vi "Add Channel Properties To String Array.vi"(8 "error in":errorcluster, 10 "Properties List In":string[][](array[string]), 11 "Channel Ref in":T1 format="%.0x") -> (0 "error out":errorcluster, 2 "Properties List Out":string[][](array[string]), 3 "Channel Ref out":T1 format="%.0x")   [LabVIEW 2026, in "SEECD System Explorer.lvlib"]
uses:
  SEECD System Explorer.lvlib
  <vilib>/NI VeriStand/Custom Device API/Custom Device Item Ref.ctl
  Shared/Type Defs/ECAT Channel Data Type.ctl
  <vilib>/Utility/error.llb/Trim Whitespace One-Sided.vi
  C:/Users/Administrator/Desktop/Jatin/All DNC DLLs/NationalInstruments.VeriStand.SystemDefinitionAPI.dll
  Jatin/All DNC DLLs/NationalInstruments.VeriStand.SystemDefinitionAPI.dll
  Shared/Globals/Property Strings.vi
  C:/Users/Administrator/Desktop/Jatin/All DNC DLLs/NationalInstruments.VeriStand.SystemStorage.dll
  Jatin/All DNC DLLs/NationalInstruments.VeriStand.SystemStorage.dll
  Shared/SEECD Shared.lvlib
  <vilib>/NI VeriStand/Custom Device API/Custom Device API.lvlib
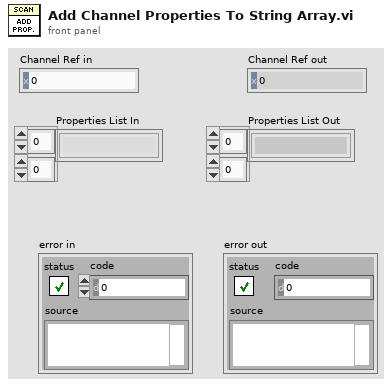
[diagram p1: front panel]
types:
  T1 = typedef "Custom Device API.lvlib/Custom Device Item Ref.ctl" = u64
  T2 = typedef "SEECD Shared.lvlib/ECAT Channel Data Type.ctl" = enum16{"Boolean", "Fixed Point", "Int8", "Int16", "Int32", "Int64", "U32 Bit Field", "UInt8", "UInt16", "UInt32", "UInt64", "Other", "DBL", "SGL"}
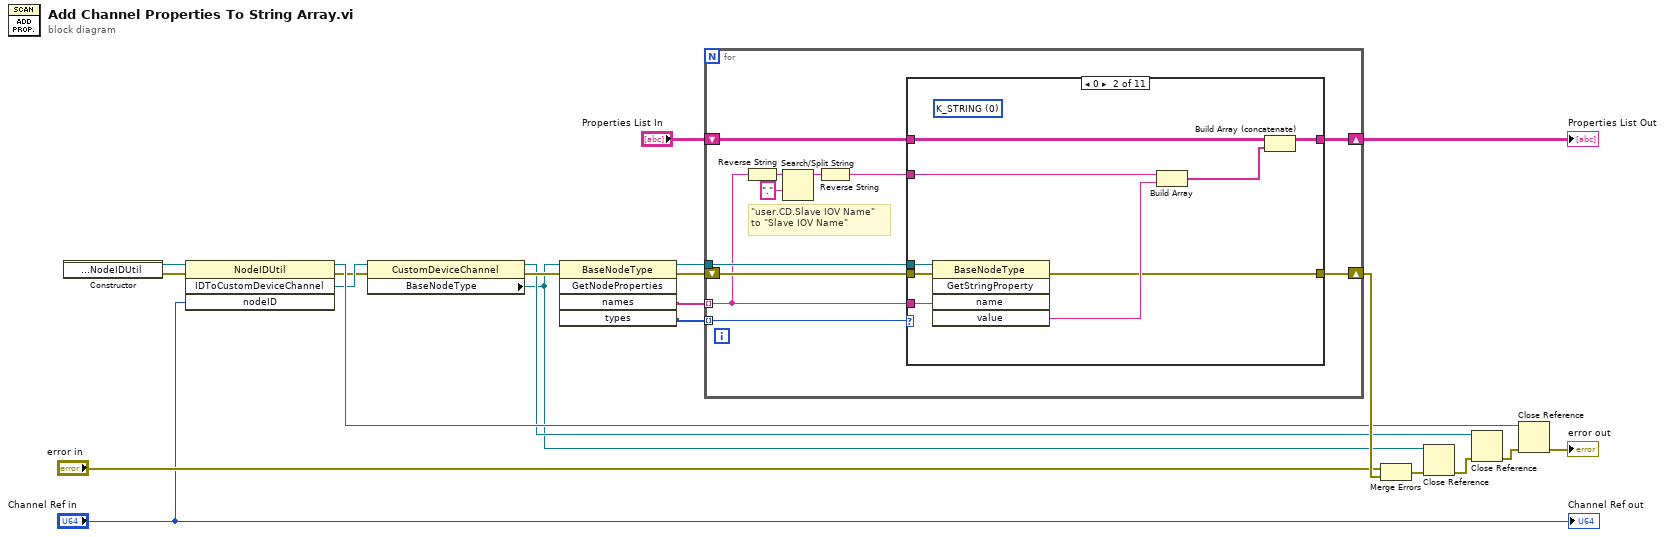
[diagram p0: block diagram]
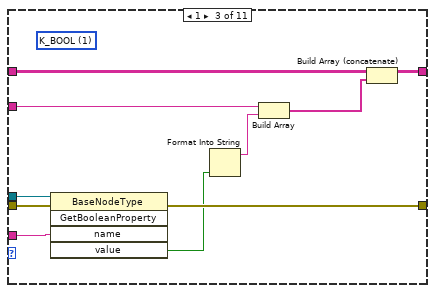
[diagram p3: hidden frame]
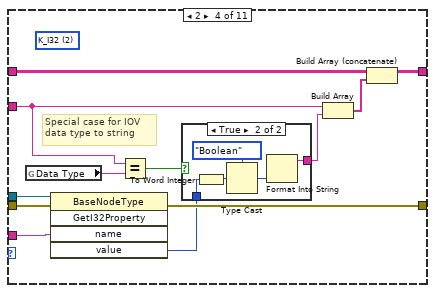
[diagram p4: hidden frame]
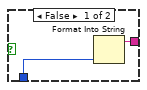
[diagram p5: hidden frame]
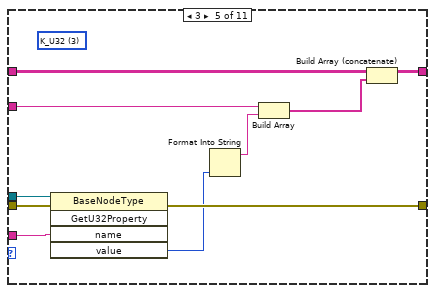
[diagram p6: hidden frame]
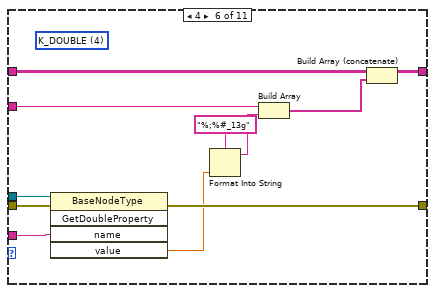
[diagram p7: hidden frame]
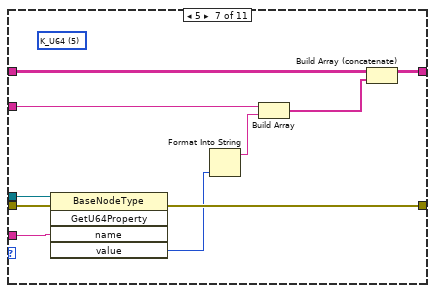
[diagram p8: hidden frame]
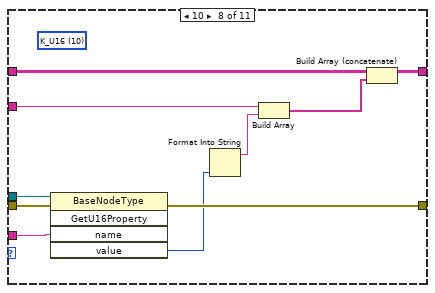
[diagram p9: hidden frame]
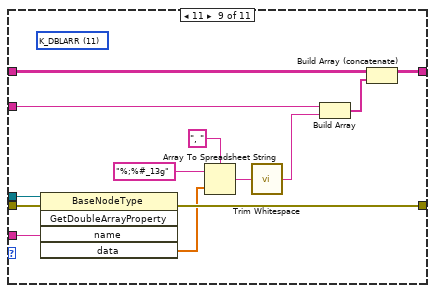
[diagram p10: hidden frame]
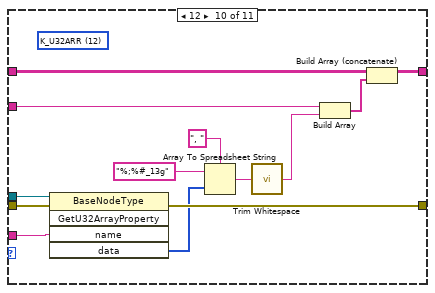
[diagram p11: hidden frame]
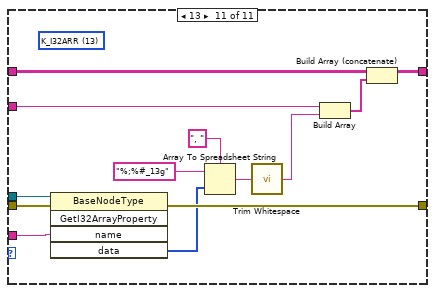
[diagram p12: hidden frame]
diagram:
  n1 = constructor class="NodeIDUtil"() -> (reference out=w14:refnum<k39>, error out=w13:errorcluster)  [unwired: 3 in, 1 out]
  n2 = invoke class="NodeIDUtil" method="IDToCustomDeviceChannel"(reference=w14, error in=w13, "nodeID"="Channel Ref in") -> (reference out=w12:refnum<k39>, error out=w10:errorcluster, "IDToCustomDeviceChannel"=w11:refnum<k39>)  [unwired: 1 in, 1 out]
  n3 = property class="CustomDeviceChannel"(reference=w11, error in=w10) -> (reference out=w8:refnum<k39>, error out=w9:errorcluster, "BaseNodeType"=w3:refnum<k39>)
  n4 = invoke class="BaseNodeType" method="GetNodeProperties"(reference=w3, error in=w9) -> (reference out=w20:refnum<k39>, error out=w15:errorcluster, "names"=w19:string[], "types"=w21:i32[])  [unwired: 3 in, 1 out]
  n5 = for {
    shift-right: [w30] -> w18
    shift-left: w15 -> [w28]
    tunnel: w19 -> [w23] mode=indexing
    shift-right: [w32] -> w17
    shift-left: "Properties List In" -> [w31]
    tunnel: w21 -> [w22] mode=indexing
    tunnel: w20 -> [w29]
    # "\"user.CD.Slave IOV Name\"\nto \"Slave IOV Name\""
    n6 = Reverse String(1:w23) -> (0:w27:string)
    n7 = Search/Split String(string=w27, search string/char (-)=".") -> (substring before match=w26:string)  [unwired: 1 in, 2 out]
    n8 = Reverse String(1:w26) -> (0:w24:string)
    n9 = case shown="0" w22 {
      tunnel: [w34 w37 w48 w61 w77 w88 w98 w108 w121 w134 w147] -> w32
      tunnel: w31 -> [w34 w43 w53 w65 w82 w93 w103 w113 w126 w139 w152]
      tunnel: [w33 w38 w49 w62 w78 w89 w99 w109 w122 w135 w148] -> w30
      tunnel: w23 -> [_ w40 w50 w57 w79 w90 w100 w110 w123 w136 w149]
      tunnel: w29 -> [_ w42 w52 w64 w81 w92 w102 w112 w125 w138 w151]
      tunnel: w28 -> [w33 w41 w51 w63 w80 w91 w101 w111 w124 w137 w150]
      tunnel: w24 -> [_ w35 w44 w55 w73 w83 w94 w104 w114 w127 w140]
      frame Default {
      }
      frame 0 {
        (unwired) 0 items=["K_STRING", "K_BOOL", "K_I32", "K_U32", "K_DOUBLE", "K_U64", "K_VARIANT", "K_DEPENDENTFILE", "K_DEPENDENTNODE", "K_DATASOURCENODE", "K_U16", "K_DBLARR", "K_U32ARR", "K_I32ARR"]
        n10 = invoke class="BaseNodeType" method="GetStringProperty"(reference=w42, error in=w41, "name"=w40) -> (error out=w38:errorcluster, "value"=w39:string)  [unwired: 2 in, 3 out]
        n11 = Build Array(w35, w39) -> (w36:string[])
        n12 = Build Array (concatenate)(w43, w36) -> (w37:string[][])
      }
      frame 1 {
        (unwired) 1 items=["K_STRING", "K_BOOL", "K_I32", "K_U32", "K_DOUBLE", "K_U64", "K_VARIANT", "K_DEPENDENTFILE", "K_DEPENDENTNODE", "K_DATASOURCENODE", "K_U16", "K_DBLARR", "K_U32ARR", "K_I32ARR"]
        n13 = invoke class="BaseNodeType" method="GetBooleanProperty"(reference=w52, error in=w51, "name"=w50) -> (error out=w49:errorcluster, "value"=w46:bool)  [unwired: 2 in, 3 out]
        n14 = Format Into String(w46) -> (resulting string=w45:string)  [unwired: 3 in, 1 out]
        n15 = Build Array(w44, w45) -> (w47:string[])
        n16 = Build Array (concatenate)(w53, w47) -> (w48:string[][])
      }
      frame 2 {
        (unwired) 2 items=["K_STRING", "K_BOOL", "K_I32", "K_U32", "K_DOUBLE", "K_U64", "K_VARIANT", "K_DEPENDENTFILE", "K_DEPENDENTNODE", "K_DATASOURCENODE", "K_U16", "K_DBLARR", "K_U32ARR", "K_I32ARR"]
        # "Special case for IOV data type to string"
        n17 = global read "Property Strings.vi" "Data Type"() -> (w56:string)
        n18 = invoke class="BaseNodeType" method="GetI32Property"(reference=w64, error in=w63, "name"=w57) -> (error out=w62:errorcluster, "value"=w59:i32)  [unwired: 2 in, 3 out]
        n19 = Equal?(x=w55, y=w56) -> (x = y?=w58:bool)
        n20 = case shown="True" w58 {
          tunnel: w59 -> [w67 w70]
          tunnel: [w66 w68] -> w54
          frame False {
            n21 = Format Into String(w67) -> (resulting string=w66:string)  [unwired: 3 in, 1 out]
          }
          frame True {
            n22 = To Word Integer(number=w70) -> (16bit integer=w72:i16)
            n23 = Type Cast(type=ECAT_Channel_Data_Type."Boolean" ("UDV Data Type"), x=w72) -> (*(type *) &x=w69:T2)
            n24 = Format Into String(w69) -> (resulting string=w68:string)  [unwired: 3 in, 1 out]
          }
        }
        n25 = Build Array(w55, w54) -> (w60:string[])
        n26 = Build Array (concatenate)(w65, w60) -> (w61:string[][])
      }
      frame 3 {
        (unwired) 3 items=["K_STRING", "K_BOOL", "K_I32", "K_U32", "K_DOUBLE", "K_U64", "K_VARIANT", "K_DEPENDENTFILE", "K_DEPENDENTNODE", "K_DATASOURCENODE", "K_U16", "K_DBLARR", "K_U32ARR", "K_I32ARR"]
        n27 = invoke class="BaseNodeType" method="GetU32Property"(reference=w81, error in=w80, "name"=w79) -> (error out=w78:errorcluster, "value"=w75:u32)  [unwired: 2 in, 3 out]
        n28 = Format Into String(w75) -> (resulting string=w74:string)  [unwired: 3 in, 1 out]
        n29 = Build Array(w73, w74) -> (w76:string[])
        n30 = Build Array (concatenate)(w82, w76) -> (w77:string[][])
      }
      frame 4 {
        (unwired) 4 items=["K_STRING", "K_BOOL", "K_I32", "K_U32", "K_DOUBLE", "K_U64", "K_VARIANT", "K_DEPENDENTFILE", "K_DEPENDENTNODE", "K_DATASOURCENODE", "K_U16", "K_DBLARR", "K_U32ARR", "K_I32ARR"]
        n31 = invoke class="BaseNodeType" method="GetDoubleProperty"(reference=w92, error in=w91, "name"=w90) -> (error out=w89:errorcluster, "value"=w86:dbl)  [unwired: 2 in, 3 out]
        n32 = Format Into String(format string="%;%#_13g", w86) -> (resulting string=w85:string)  [unwired: 2 in, 1 out]
        n33 = Build Array(w83, w85) -> (w87:string[])
        n34 = Build Array (concatenate)(w93, w87) -> (w88:string[][])
      }
      frame 5 {
        (unwired) 5 items=["K_STRING", "K_BOOL", "K_I32", "K_U32", "K_DOUBLE", "K_U64", "K_VARIANT", "K_DEPENDENTFILE", "K_DEPENDENTNODE", "K_DATASOURCENODE", "K_U16", "K_DBLARR", "K_U32ARR", "K_I32ARR"]
        n35 = invoke class="BaseNodeType" method="GetU64Property"(reference=w102, error in=w101, "name"=w100) -> (error out=w99:errorcluster, "value"=w96:u64)  [unwired: 2 in, 3 out]
        n36 = Format Into String(w96) -> (resulting string=w95:string)  [unwired: 3 in, 1 out]
        n37 = Build Array(w94, w95) -> (w97:string[])
        n38 = Build Array (concatenate)(w103, w97) -> (w98:string[][])
      }
      frame 10 {
        (unwired) 10 items=["K_STRING", "K_BOOL", "K_I32", "K_U32", "K_DOUBLE", "K_U64", "K_VARIANT", "K_DEPENDENTFILE", "K_DEPENDENTNODE", "K_DATASOURCENODE", "K_U16", "K_DBLARR", "K_U32ARR", "K_I32ARR"]
        n39 = invoke class="BaseNodeType" method="GetU16Property"(reference=w112, error in=w111, "name"=w110) -> (error out=w109:errorcluster, "value"=w106:u16)  [unwired: 2 in, 3 out]
        n40 = Format Into String(w106) -> (resulting string=w105:string)  [unwired: 3 in, 1 out]
        n41 = Build Array(w104, w105) -> (w107:string[])
        n42 = Build Array (concatenate)(w113, w107) -> (w108:string[][])
      }
      frame 11 {
        (unwired) 11 items=["K_STRING", "K_BOOL", "K_I32", "K_U32", "K_DOUBLE", "K_U64", "K_VARIANT", "K_DEPENDENTFILE", "K_DEPENDENTNODE", "K_DATASOURCENODE", "K_U16", "K_DBLARR", "K_U32ARR", "K_I32ARR"]
        n43 = invoke class="BaseNodeType" method="GetDoubleArrayProperty"(reference=w125, error in=w124, "name"=w123) -> (error out=w122:errorcluster, "data"=w119:dbl[])  [unwired: 2 in, 3 out]
        n44 = Array To Spreadsheet String(delimiter (Tab)=", ", array=w119, 3:"%;%#_13g" ("format string")) -> (spreadsheet string=w118:string)
        n45 = call <vilib>:"Trim Whitespace.vi"("string"=w118) -> ("trimmed string"=w117:string)  [unwired: 1 in]
        n46 = Build Array(w114, w117) -> (w120:string[])
        n47 = Build Array (concatenate)(w126, w120) -> (w121:string[][])
      }
      frame 12 {
        (unwired) 12 items=["K_STRING", "K_BOOL", "K_I32", "K_U32", "K_DOUBLE", "K_U64", "K_VARIANT", "K_DEPENDENTFILE", "K_DEPENDENTNODE", "K_DATASOURCENODE", "K_U16", "K_DBLARR", "K_U32ARR", "K_I32ARR"]
        n48 = invoke class="BaseNodeType" method="GetU32ArrayProperty"(reference=w138, error in=w137, "name"=w136) -> (error out=w135:errorcluster, "data"=w132:u32[])  [unwired: 2 in, 3 out]
        n49 = Array To Spreadsheet String(delimiter (Tab)=", ", array=w132, 3:"%;%#_13g" ("format string")) -> (spreadsheet string=w131:string)
        n50 = call <vilib>:"Trim Whitespace.vi"("string"=w131) -> ("trimmed string"=w130:string)  [unwired: 1 in]
        n51 = Build Array(w127, w130) -> (w133:string[])
        n52 = Build Array (concatenate)(w139, w133) -> (w134:string[][])
      }
      frame 13 {
        (unwired) 13 items=["K_STRING", "K_BOOL", "K_I32", "K_U32", "K_DOUBLE", "K_U64", "K_VARIANT", "K_DEPENDENTFILE", "K_DEPENDENTNODE", "K_DATASOURCENODE", "K_U16", "K_DBLARR", "K_U32ARR", "K_I32ARR"]
        n53 = invoke class="BaseNodeType" method="GetI32ArrayProperty"(reference=w151, error in=w150, "name"=w149) -> (error out=w148:errorcluster, "data"=w145:i32[])  [unwired: 2 in, 3 out]
        n54 = Array To Spreadsheet String(delimiter (Tab)=", ", array=w145, 3:"%;%#_13g" ("format string")) -> (spreadsheet string=w144:string)
        n55 = call <vilib>:"Trim Whitespace.vi"("string"=w144) -> ("trimmed string"=w143:string)  [unwired: 1 in]
        n56 = Build Array(w140, w143) -> (w146:string[])
        n57 = Build Array (concatenate)(w152, w146) -> (w147:string[][])
      }
    }
  }
  "Properties List Out" <- w17
  n58 = Merge Errors("error in", w18) -> (w2:errorcluster)
  n59 = Close Reference(reference=w3, error in (no error)=w2) -> (error out=w4:errorcluster)
  n60 = Close Reference(reference=w8, error in (no error)=w4) -> (error out=w7:errorcluster)
  n61 = Close Reference(reference=w12, error in (no error)=w7) -> (error out=→"error out":errorcluster)
  "Channel Ref out" <- "Channel Ref in"
